vi "Init.vi"(8 "error in (no error)":errorcluster, 11 "Simulated Videocamera in":refnum<class "Simulated Videocamera.lvclass">) -> (0 "error out":errorcluster, 3 "Simulated Videocamera out":refnum<class "Simulated Videocamera.lvclass">)   [LabVIEW 2014, in "Simulated Videocamera.lvclass"]
uses:
  Simulated Videocamera.lvclass
  Framework/Model/Data/Data2D/Data2D.lvclass
  Simulated Videocamera.lvclass/Simulated Videocamera.ctl
  <vilib>/Utility/file.llb/Read From Spreadsheet File (DBL).vi
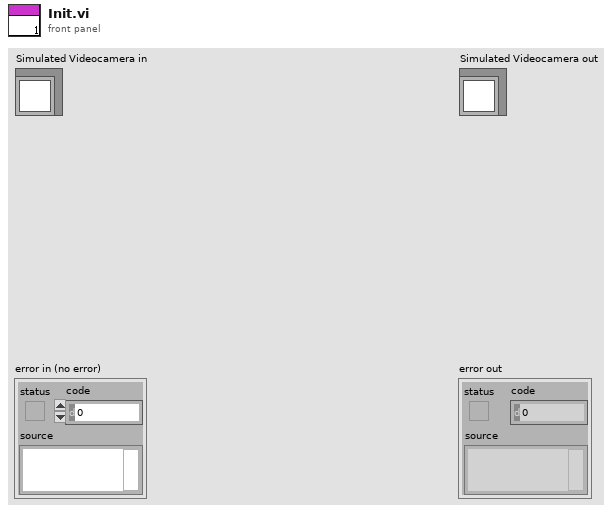
[diagram p1: front panel]
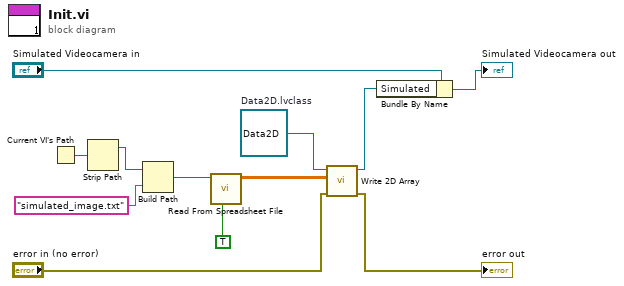
[diagram p0: block diagram]
diagram:
  w2 = refnum<class "Data2D.lvclass"> refnum  # Data2D.lvclass
  n1 = Current VI's Path() -> (path=w12:path)
  n2 = Strip Path(path=w12) -> (stripped path=w11:path)  [unwired: 1 out]
  n3 = Build Path(base path=w11, name or relative path="simulated_image.txt") -> (appended path=w9:path)
  n4 = call-poly <vilib>:"Read From Spreadsheet File.vi"("transpose (no:F)"=TRUE, "file path (dialog if empty)"=w9) -> ("all rows"=w6:dbl[][])  [unwired: 5 in, 4 out]
  n5 = call "Write 2D Array.vi"("error in (no error)"="error in (no error)", "2D Array"=w6, "Data2D in"=w2) -> ("error out"=→"error out":errorcluster, "Data2D out"=w5:refnum<class "Data2D.lvclass">)  [unwired: 7 in]
  n6 = Bundle By Name(cluster="Simulated Videocamera in", "Simulated"=w5) -> (→"Simulated Videocamera out":refnum<class "Simulated Videocamera.lvclass">)
